vi "GetState_Video.vi"(8 "error in (no error)":errorcluster, 11 "VLC Variables In":T2) -> (0 "error out":errorcluster, 1 "State":T1=1 items=["IDLE/CLOSE", "OPENING", "BUFFERING", "PLAYING", "PAUSED", "STOPPING", "ENDED", "ERROR"], 3 "VLC Variables Out":T2)   [LabVIEW 2012]
doc: "Get the state of the video, the state can be: Idle, opening, buffering, playing, paused, stoping or ended."
uses:
  Controls-Webcam/VLC Var.ctl
  Controls-Webcam/VLC State.ctl
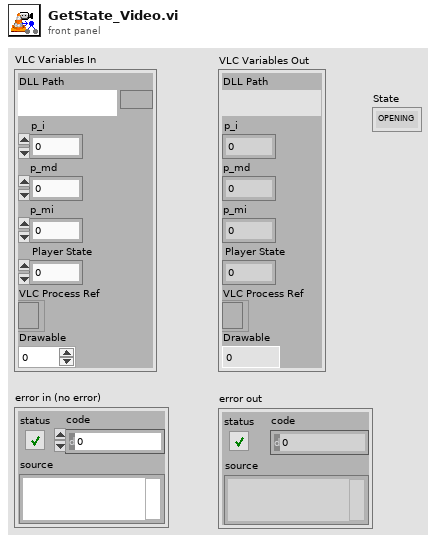
[diagram p1: front panel]
types:
  T1 = typedef "VLC State.ctl" = i32
  T2 = typedef "VLC Var.ctl" = cluster{"DLL Path":path, "p_i":i32, "p_md":i32, "p_mi":i32, "Player State":i32, "VLC Process Ref":refnum<k24>, "Drawable":i32}
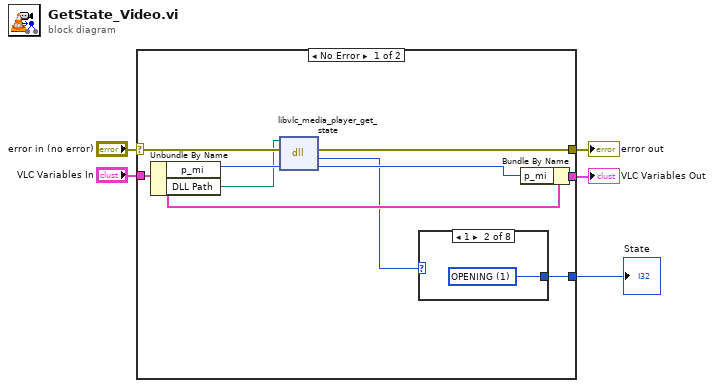
[diagram p0: block diagram]
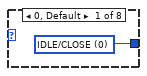
[diagram p2: hidden frame]
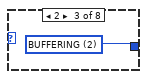
[diagram p3: hidden frame]
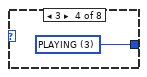
[diagram p4: hidden frame]
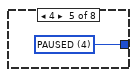
[diagram p5: hidden frame]
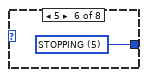
[diagram p6: hidden frame]
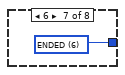
[diagram p7: hidden frame]
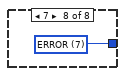
[diagram p8: hidden frame]
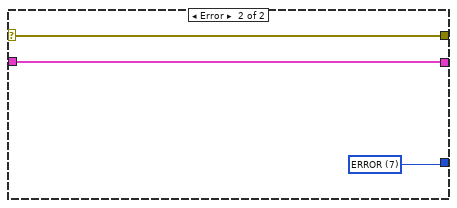
[diagram p9: hidden frame]
diagram:
  n1 = case shown="No Error" "error in (no error)" {
    selector: "error in (no error)" -> [w8 w25]
    tunnel: [w14 w24] -> w5
    tunnel: "VLC Variables In" -> [w11 w24]
    tunnel: [w10 w25] -> w3
    tunnel: [w7 w23] -> w1
    frame No Error {
      n2 = Unbundle By Name(w11) -> ("p_mi"=w12:i32, "DLL Path"=w6:path)
      n3 = dll-call lib="C:/Program Files (x86)/VideoLAN/VLC/libvlc.dll" fn="libvlc_media_player_get_state"(path in=w6, error in=w8, "p_mi"=w12) -> (error out=w10:errorcluster, "return type"=w9:i32, "p_mi"=w13:i32)  [unwired: 1 in, 1 out]
      n4 = case shown="1" w9 {
        tunnel: [w15 w16 w17 w18 w19 w20 w21 w22] -> w7
        frame 0, Default {
          w15 = T1 0 items=["IDLE/CLOSE", "OPENING", "BUFFERING", "PLAYING", "PAUSED", "STOPPING", "ENDED", "ERROR"] ("State 2")
        }
        frame 1 {
          w16 = T1 1 items=["IDLE/CLOSE", "OPENING", "BUFFERING", "PLAYING", "PAUSED", "STOPPING", "ENDED", "ERROR"] ("State 2")
        }
        frame 2 {
          w17 = T1 2 items=["IDLE/CLOSE", "OPENING", "BUFFERING", "PLAYING", "PAUSED", "STOPPING", "ENDED", "ERROR"] ("State 2")
        }
        frame 3 {
          w18 = T1 3 items=["IDLE/CLOSE", "OPENING", "BUFFERING", "PLAYING", "PAUSED", "STOPPING", "ENDED", "ERROR"] ("State 2")
        }
        frame 4 {
          w19 = T1 4 items=["IDLE/CLOSE", "OPENING", "BUFFERING", "PLAYING", "PAUSED", "STOPPING", "ENDED", "ERROR"] ("State 2")
        }
        frame 5 {
          w20 = T1 5 items=["IDLE/CLOSE", "OPENING", "BUFFERING", "PLAYING", "PAUSED", "STOPPING", "ENDED", "ERROR"] ("State 2")
        }
        frame 6 {
          w21 = T1 6 items=["IDLE/CLOSE", "OPENING", "BUFFERING", "PLAYING", "PAUSED", "STOPPING", "ENDED", "ERROR"] ("State 2")
        }
        frame 7 {
          w22 = T1 7 items=["IDLE/CLOSE", "OPENING", "BUFFERING", "PLAYING", "PAUSED", "STOPPING", "ENDED", "ERROR"] ("State 2")
        }
      }
      n5 = Bundle By Name(cluster=w11, "p_mi"=w13) -> (w14:T2)
    }
    frame Error {
      w23 = T1 7 items=["IDLE/CLOSE", "OPENING", "BUFFERING", "PLAYING", "PAUSED", "STOPPING", "ENDED", "ERROR"] ("State 2")
    }
  }
  "VLC Variables Out" <- w5
  "error out" <- w3
  "State" <- w1
